vi "Digilens DLP Gen2 UI .vi"(11 "TopLevel In":refnum<class "TopLevel.lvclass">) -> (3 "TopLevel Out":refnum<class "TopLevel.lvclass">)   [LabVIEW 2022 SP3, in "TopLevel.lvclass"]
uses:
  TopLevel.lvclass
  Typedefs/SettinsgTabs--Tab.ctl
  Icons/Load.ctl
  Icons/HeadButton.ctl
  Icons/Enable.ctl
  Icons/go_button.ctl
  Typedefs/AdvPrinterControl--Tabs.ctl
  Common/Controls/ImageResolution--enum.ctl
  Icons/GreenControl_64.ctl
  GIS Printer/Typedefs/Print Types.ctl
  Typedefs/MainTabs--tabs.ctl
  Typedefs/Dummy--Tabs.ctl
  Typedefs/PurgeMode--Enum.ctl
  Typedefs/processMode--enum.ctl
  DAQWFE/LV_Source/Subsystems/DAQ/DAQ.lvclass
  <vilib>/TELLC/Dynamic CVT API/TD Dynamic CVT DVR--ref.ctl
  DAQWFE/LV_Source/Subsystems/DAQ/DataTypes/TD DAQ DI state change ev.ctl
  Typedefs/UserLevel_withoutNone--Enum.ctl
  DAQ_Common/DataTypes/TD IOCtrlUpdate.ctl
  DLP2/DLP2.lvclass/DLP2.ctl
  Typedefs/PrinterHeads--Enum.ctl
  Motor Controller/Typedefs/API Command Cluster.ctl
  Motor Controller/Typedefs/API Command Enum.ctl
  Motor Controller/Typedefs/SetExplicitMessage API Data.ctl
  Motor Controller/Typedefs/Motor Controller Parameter-Set.ctl
  IO/Typedefs/ICP1-D0 Channel Names.ctl
  Typedefs/HeadPrintData--Cluster.ctl
  Motor Controller/Typedefs/Motor Controller Parameter-Get.ctl
  Typedefs/API Command Enum.ctl
  Typedefs/PrimingMode APIData.ctl
  Typedefs/API Command Cluster.ctl
  GIS Printer/Typedefs/PrintCmdParameters--Cluster.ctl
  GIS Printer/Typedefs/IdlePrintCmdParameters--Cluster.ctl
  IO/Typedefs/ICP2-DO Channel Names.ctl
  GIS Printer/GIS Printer.lvclass/GIS Printer.ctl
  Common/Controls/RecipeInfo--Cluster.ctl
  Common/Controls/DLP RecipeTypesData--Cluster.ctl
  IO/IO.lvclass
  GIS Printer/GIS Printer.lvclass
  Motor Controller/Motor Controller.lvclass
  Motor Controller/Typedefs/Status.ctl
  Typedefs/Motor Controller Config Data.ctl
  Motor Controller/Typedefs/Stage Move Data.ctl
  Motor Controller/Typedefs/Batch Index Speed Data.ctl
  Motor Controller/Typedefs/Move Status.ctl
  IO/Typedefs/Pre Purge Parameters.ctl
  Database/Database.lvclass
  DLP2/DLP2.lvclass
  Common/Controls/TD MasterConfiguration DLPC2--cluster.ctl
  Common/Controls/DLPC2_Path--Cluster.ctl
  Common/Controls/TD HeadColorPaneMappingAll--cluster.ctl
  Common/Controls/TD HeadColorPaneMapping--cluster.ctl
  Typedefs/SpitVoltages--Cluster.ctl
  <vilib>/vision/Image Controls.llb/IMAQ Image.ctl
  Typedefs/TiffImageData--Cluster.ctl
  Common/Controls/Imageresolution--cluster.ctl
  GIS Printer/Typedefs/GIS Status--Cluster.ctl
  GIS Printer/Typedefs/HeadEnableStatus--cluster.ctl
  DLP2/DataTypes/SeperateLayersPython--cluster.ctl
  Common/Controls/PythonVersion--Enum.ctl
  Common/Controls/DLPConfig_RecipePrints.ctl
  Common/Controls/DLPConfig_CalibrationPrints.ctl
  Typedefs/LoginEventData--CLuster.ctl
  Typedefs/UserLevel--Enum.ctl
  Typedefs/printWeights--cluster.ctl
  DLP2/DataTypes/DLP2_PrinterHeadProperties.ctl
  Common/Controls/DLPConfig)Init_HeadPropertyAttr--Cluster.ctl
  Common/Controls/DLP_MaterialToHeadMapping--Cluster.ctl
  DLP2/DataTypes/DLP2_PrinterMaterialProperties.ctl
  Typedefs/InkIdleNodeConfigXML--Cluster.ctl
  IO/Typedefs/Status Cluster.ctl
  IO/Typedefs/ICP2-DI Channel Names.ctl
  IO/Typedefs/ICP1-AI Channel Names.ctl
  IO/Typedefs/ICP1-AO Channel Names.ctl
  IO/Typedefs/ICP2-AO Channel Names.ctl
  Motor Controller/Typedefs/Status_TopLevel--Cluster.ctl
  DLP2/DataTypes/LoadImagesData--cluster.ctl
  Common/Controls/RecipesFolderSummary--Cluster.ctl
  <vilib>/Analysis/baseanly.llb/Mean (DBL).vi
  DLP2/Accessors/Get PublicEvents.vi
  DAQWFE/LV_Source/DataTypes/GBL System.vi
  <vilib>/Utility/config.llb/Write Key (Path).vi
  GIS Printer/Methods/Variant_To_DVR.vi
  <userlib>/_OpenG.lib/array/array.llb/Sort 1D Array (I32)__ogtk.vi
  <vilib>/Analysis/NI_AALBase.lvlib
  <vilib>/Utility/config.llb/NI_LVConfig.lvlib
  <vilib>/vision/NI_Vision_Development_Module.lvlib
panel:
  in  "General":bool
  in  "CALIBRATION RECIPE XML FOLDER PATH":path
  in  "INITIALIZATION FILE PATH":path
  in  "PRODUCT RECIPE XML FOLDER PATH":path
  in  "Head 1 ColorPlane":u16(ring) items=["1", "0", "3", "2", "None", "None2"]
  in  "Head 2 ColorPlane":u16(ring) items=["1", "0", "3", "2", "None", "None2"]
  in  "Head 3 ColorPlane":u16(ring) items=["1", "0", "3", "2", "None", "None2"]
  in  "Head 4 ColorPlane":u16(ring) items=["1", "0", "3", "2", "None", "None2"]
  in  "Head 5 ColorPlane":u16(ring) items=["1", "0", "3", "2", "None", "None2"]
  in  "Head 6 ColorPlane":u16(ring) items=["1", "0", "3", "2", "None", "None2"]
  out "Head 1 Material":u16(ring) items=["109G", "113A_3", "507_2(50)", "507_2", "None", "None2"]
  out "Head 2 Material":u16(ring) items=["109G", "113A_3", "507_2(50)", "507_2", "None", "None2"]
  out "Head 3 Material":u16(ring) items=["109G", "113A_3", "507_2(50)", "507_2", "None", "None2"]
  out "Head 4 Material":u16(ring) items=["109G", "113A_3", "507_2(50)", "507_2", "None", "None2"]
  out "Head 5 Material":u16(ring) items=["109G", "113A_3", "507_2(50)", "507_2", "None", "None2"]
  out "Head 6 Material":u16(ring) items=["109G", "113A_3", "507_2(50)", "507_2", "None", "None2"]
  out "PPP search string":string
  in  "LoadImages":bool
  in  "Enable Disable With DO":T1
  in  "Jog (+) 1":bool
  in  "Jog (-) 1":bool
  in  "Abort 2":bool
  in  "Home 3":bool
  in  "Stage Abort":bool
  in  "Abort":bool
  in  "Home Stg 2":bool
  in  "Jog (+) 2":bool
  in  "Jog (-) 2":bool
  in  "Home":bool
  out "NameArray":string[](array[string])
  in  "INK H 11":T2
  out "LogINDetail":string
  in  "AdvPrinterTabsBtn":bool
  out "H6 Long Idle":bool
  out "H2 Long Idle":bool
  out "H1 Long Idle":bool
  out "H3 Long Idle":bool
  out "H4 Long Idle":bool
  out "H5 Long Idle":bool
  out "H6 Short Idle":bool
  out "H2 Short Idle":bool
  out "H1 Short Idle":bool
  out "H3 Short Idle":bool
  out "H4 Short Idle":bool
  out "H5 Short Idle":bool
  out "Stage Busy (Moves)":bool caption="Stage Busy"
  in  "5Pass":bool
  in  "10Pass":bool
  in  "Login":bool
  out "H6ColorPlane":string
  out "H5ColorPlane":string
  out "H4ColorPlane":string
  out "H3ColorPlane":string
  out "H2ColorPlane":string
  out "H1ColorPlane":string
  in  "IdleMode":T3
  in  "ImageResolution":T4
  out "Resolution":string
  in  "DLP GUI Config":path
  in  "SAVE DLP Config":bool
  in  "Apply DLP GUI Config":bool
  out "Meniscus Valve Open - R1_Status 2":T3
  out "Meniscus Valve Open - R2_Status 2":T3
  out "Meniscus Valve Open - R3_Status 2":T3
  out "Meniscus Valve Open - R4_Status 2":T3
  out "Meniscus Valve Open - R5_Status 2":T3
  out "Meniscus Valve Open - R6_Status 2":T3
  in  "PrinterControlsX":T5
  out "ImageMain":T6(plugin-control)
  in  "Head6 Temp 1":string
  in  "Head5 Temp 1":string
  in  "Head4 Temp 1":string
  in  "Head3 Temp 1":string
  in  "Head2 Temp 1":string
  in  "Head1 Temp 1":string
  in  "Stage Recipe XML File Path":path
  in  "Start":bool
  in  "Stage Move Status":i32(listbox)
  in  "Idle Intervals (s)":dbl=0.1
  in  "IdlePrint":bool
  in  "StartPrintSequence":bool
  in  "Load Customer Design":bool
  in  "Print Types":T7
  out "Version":string
  out "date/time string":string
  out "Type":string
  in  "GetMat&Color":bool
  in  "PPDuration (s)":dbl=3.0
  in  "Duration (s)":dbl=3.0
  out "AI ScanArray":dbl[](array[numeric])
  in  "Exit":bool
  in  "Settings":bool
  in  "Drop Watch":bool
  in  "Stage Control":bool
  in  "Printhead Service":bool
  in  "IPLC Process":bool
  out "Stage Busy Printer":bool caption="Busy"
  out "Status/Error :":string
  out "H 6":dbl
  out "H 5":dbl
  out "H 4":dbl
  out "H 3":dbl
  out "H 2":dbl
  out "H1":dbl
  in  "Tab Control":T8
  out "PrintStatus":string
  in  "Refresh Timer":bool
  out "HeadPrimeTimer":i32
  in  "Recipe":u16(ring) items=["c30v3_1 Recipe DOE485", "c30v3_1 Recipe DOE485 Green", "c30v3_1 Recipe PORtest"]
  in  "Product":u16(ring) items=["C30v3_1", "Haze", "SingleColor1_5"]
  in  "RecipeType":u16(ring) items=["PrintDesign", "Calibration"]
  in  "PrintControlTab":enum32{"Product", "Calibration"}(tab)
  in  "Print PPP Image":bool
  in  "RIP Recipe":bool
  out "CalPrint Counter":i32
  in  "Load Calibration Rx":bool
  in  "PrintHead Number":u16(ring)=1 caption="Head" items=["1", "2", "3", "4", "5", "6"]
  in  "Head Print Command":bool
  in  "Refresh":bool
  in  "PrimeHeads":bool
  in  "AbortPrinterOperation":bool
  out "ImageMain 5":T6(plugin-control)
  out "ImageMain 3":T6(plugin-control)
  out "ImageMain 4":T6(plugin-control)
  out "ImageMain 2":T6(plugin-control)
  in  "ProcessMode":T9
  in  "Load":T10
  in  "Laminate":T10
  in  "PurgeMove H1":T11
  in  "PurgeMove H2":T11
  in  "PurgeMove H3":T11
  in  "PurgeMove H4":T11
  in  "PurgeMove H5":T11
  in  "PurgeMove H6":T11
  out "Status":string
  in  "Jog (-)":bool
  in  "Jog (+)":bool
  in  "Jog Speed":i32
  in  "Print Speed (-)":bool
  in  "Print (+)":bool
  in  "Print Speed":i32
  in  "GoTo":i32
  in  "Speed":i32
  in  "Go":T12
  out "Position":dbl
  out "Pulse/mm":dbl
  in  "Head1":T11
  in  "Head2":T11
  in  "Head3":T11
  in  "Head4":T11
  in  "Head5":T11
  in  "Head6":T11
  in  "Read Status":bool
  in  "Enable Disable":T1
  in  "ClearStageAlarm":bool
  out "Stage Enabled":bool
  out "Stage Busy (Stage)":bool caption="Stage Busy"
  in  "PrinterControls 5":T2
  in  "Weights 5":dbl=0.15 min=0.01 max=0.15
  in  "Freq 5":i32
  in  "Head 5 Material 2":u16(ring) items=["109G", "113A_3", "507_2(50)", "507_2", "None", "None2"]
  in  "Heater-5 Off 2":bool
  out "Head 5 Act Temp":dbl
  in  "Enable Ink Ch-5":bool
  in  "Head5 TempSet":dbl
  in  "Head 5 Set":bool
  in  "Prime Mode 5":T13
  in  "Prime Duration 5":dbl=0.3
  in  "Prime Interavl 5":dbl
  in  "Prime Repeats 5":u8=1 min=1
  in  "StartPrime 5":bool
  in  "Stage Head5 2":bool
  out "H5 Status":T3
  out "HH5 Status":T3
  in  "PrinterControls 4":T2
  in  "Weights 4":dbl=0.15 min=0.01 max=0.15
  in  "Freq 4":i32
  in  "Head 4 Material 2":u16(ring) items=["109G", "113A_3", "507_2(50)", "507_2", "None", "None2"]
  in  "Heater-4 Off 2":bool
  out "Head 4 Act Temp":dbl
  in  "Enable Ink Ch-4":bool
  in  "Head4 TempSet":dbl
  in  "Head 4 Set":bool
  in  "Prime Mode 4":T13
  in  "Prime Duration 4":dbl=0.3
  in  "Prime Interval 4":dbl
  in  "Prime Repeats 4":u8=1 min=1
  in  "StartPrime 4":bool
  in  "Stage Head4 2":bool
  out "H4 Status":T3
  out "HH4 Status":T3
  in  "PrinterControls 6":T2
  in  "Weights 6":dbl=0.15 min=0.01 max=0.15
  in  "Freq 6":i32
  in  "Head 6 Material 2":u16(ring) items=["109G", "113A_3", "507_2(50)", "507_2", "None", "None2"]
  in  "Heater-6 Off 2":bool
  out "Head 6 Act Temp":dbl
  in  "Enable Ink Ch-6":bool
  in  "Head6 TempSet":dbl
  in  "Head 6 Set":bool
  in  "Prime Mode 6":T13
  in  "Prime Duration 6":dbl=0.3
  in  "Prime Interval 6":dbl
  in  "Prime Repeats 6":u8=1 min=1
  in  "StartPrime 6":bool
  in  "Stage Head6 2":bool
  out "H6 Status":T3
  out "HH6 Status":T3
  in  "PrinterControls 2":T2
  in  "Weights 2":dbl=0.15 min=0.01 max=0.15
  in  "Freq 2":i32=1
  in  "Head 2 Material 2":u16(ring) items=["109G", "113A_3", "507_2(50)", "507_2", "None", "None2"]
  in  "Heater-2 Off 2":bool
  out "Head 2 Act Temp":dbl
  in  "Enable Ink Ch-2":bool
  in  "Head2 TempSet":dbl
  in  "Head 2 Set":bool
  in  "StartPrime 2":bool
  in  "Prime Mode 2":T13
  in  "Prime Duration 2":dbl=0.3
  in  "Prime Interval 2":dbl=1.0
  in  "Prime Repeats 2":u8=1 min=1
  in  "Stage Head2 2":bool
  out "H2 Status":T3
  out "HH2 Status":T3
  in  "PrinterControls 3":T2
  in  "Weights 3":dbl=0.15 min=0.01 max=0.15
  in  "Freq 3":i32
  in  "Head 3 Material 2":u16(ring) items=["109G", "113A_3", "507_2(50)", "507_2", "None", "None2"]
  in  "Heater-3 Off 2":bool
  out "Head 3 Act Temp":dbl
  in  "Enable Ink Ch-3":bool
  in  "Head3 TempSet":dbl
  in  "Head 3 Set":bool
  in  "Prime Mode 3":T13
  in  "Prime Duration 3":dbl=0.3
  in  "Prime Interval 3":dbl
  in  "Prime Repeats 3":u8=1 min=1
  in  "StartPrime 3":bool
  in  "Stage Head3 2":bool
  out "H3 Status":T3
  out "HH3 Status":T3
  in  "PrinterControls":T2
  in  "Weights 1":dbl=0.15 min=0.01 max=0.15
  in  "Freq 1":i32=1
  in  "Head 1 Material 2":u16(ring) items=["109G", "113A_3", "507_2(50)", "507_2", "None", "None2"]
  in  "Heater-1 Off 2":bool
  in  "Enable Ink Ch-1":bool
  in  "Head1 TempSet":dbl
  in  "Head 1 Set":bool
  in  "Prime Mode 1":T13
  in  "Prime Duration 1":dbl=0.3
  in  "Prime Interval 1":dbl=1.0
  in  "Prime Repeats 1":u8=1 min=1
  in  "StartPrime 1":bool
  out "Head 1 Act Temp":dbl
  in  "Stage Head1 2":bool
  out "H1 Status":T3
  out "HH1 Status":T3
  in  "SaveINIXML":bool
  out "Counts":i32
  in  "Script CMD":bool
  in  "Digital IO":bool
  in  "Analog IO":bool
  out "SettingsTabs":T14
  out "SW - Ink Valve - R2":bool
  out "SW - Ink Valve - R1":bool
  out "SW - Ink Valve - R3":bool
  out "SW - Ink Valve - R4":bool
  out "SW - Ink Valve - R5":bool
  out "SW - Ink Valve - R6":bool
  out "SW - COVER INPUT SIDE":bool
  out "SW - COVER OUTPUT SIDE":bool
  out "SW - Purge - R2":bool
  out "SW - Purge - R1":bool
  out "SW - Purge - R3":bool
  out "SW - Purge - R4":bool
  out "SW - Purge - R5":bool
  out "SW - Purge - R6":bool
  in  "Dig H 1":T2
  in  "Meniscus Pressure Reg PWR - R1":bool
  in  "SW_LED - Ink Valve - R1":bool
  in  "Meniscus Valve Open - R1":bool
  out "Meniscus Valve Open - R1_Status":T3
  out "SW_LED - Ink Valve - R1_Status":T3
  out "Meniscus Pressure Reg PWR - R1_Status":T3
  in  "Dig H 2":T2
  in  "Meniscus Pressure Reg PWR - R2":bool
  in  "SW_LED - Ink Valve - R2":bool
  in  "Meniscus Valve Open - R2":bool
  out "Meniscus Pressure Reg PWR - R2_Status":T3
  out "SW_LED - Ink Valve - R2_Status":T3
  out "Meniscus Valve Open - R2_Status":T3
  in  "Dig H 3":T2
  in  "Meniscus Pressure Reg PWR - R3":bool
  in  "SW_LED - Ink Valve - R3":bool
  in  "Meniscus Valve Open - R3":bool
  out "Meniscus Pressure Reg PWR - R3_Status":T3
  out "SW_LED - Ink Valve - R3_Status":T3
  out "Meniscus Valve Open - R3_Status":T3
  in  "Dig H 4":T2
  in  "Meniscus Pressure Reg PWR - R4":bool
  in  "SW_LED - Ink Valve - R4":bool
  in  "Meniscus Valve Open - R4":bool
  out "Meniscus Pressure Reg PWR - R4_Status":T3
  out "SW_LED - Ink Valve - R4_Status":T3
  out "Meniscus Valve Open - R4_Status":T3
  in  "Dig H 5":T2
  in  "Meniscus Pressure Reg PWR - R5":bool
  in  "SW_LED - Ink Valve - R5":bool
  in  "Meniscus Valve Open - R5":bool
  out "Meniscus Pressure Reg PWR - R5_Status":T3
  out "SW_LED - Ink Valve - R5_Status":T3
  out "Meniscus Valve Open - R5_Status":T3
  in  "Dig H 6":T2
  in  "Meniscus Pressure Reg PWR - R6":bool
  in  "SW_LED - Ink Valve - R6":bool
  in  "Meniscus Valve Open - R6":bool
  out "Meniscus Pressure Reg PWR - R6_Status":T3
  out "SW_LED - Ink Valve - R6_Status":T3
  out "Meniscus Valve Open - R6_Status":T3
  in  "INK H 6":T2
  in  "Purge Valve Open - R6":bool
  in  "Recirc Pump On - R6":bool
  in  "Ink Flow Valve Open - R6":bool
  out "Purge Valve Open - R6_Status":T3
  out "Recirc Pump On - R6_Status":T3
  out "Ink Flow Valve Open - R6_Status":T3
  in  "INK H 5":T2
  in  "Purge Valve Open - R5":bool
  in  "Recirc Pump On - R5":bool
  in  "Ink Flow Valve Open - R5":bool
  out "Purge Valve Open - R5_Status":T3
  out "Recirc Pump On - R5_Status":T3
  out "Ink Flow Valve Open - R5_Status":T3
  in  "INK H 4":T2
  in  "Purge Valve Open - R4":bool
  in  "Recirc Pump On - R4":bool
  in  "Ink Flow Valve Open - R4":bool
  out "Purge Valve Open - R4_Status":T3
  out "Recirc Pump On - R4_Status":T3
  out "Ink Flow Valve Open - R4_Status":T3
  in  "INK H 3":T2
  in  "Purge Valve Open - R3":bool
  in  "Recirc Pump On - R3":bool
  in  "Ink Flow Valve Open - R3":bool
  out "Purge Valve Open - R3_Status":T3
  out "Recirc Pump On - R3_Status":T3
  out "Ink Flow Valve Open - R3_Status":T3
  in  "INK H 2":T2
  in  "Purge Valve Open - R2":bool
  in  "Recirc Pump On - R2":bool
  in  "Ink Flow Valve Open - R2":bool
  out "Purge Valve Open - R2_Status":T3
  out "Recirc Pump On - R2_Status":T3
  out "Ink Flow Valve Open - R2_Status":T3
  in  "INK H 1":T2
  in  "Purge Valve Open - R1":bool
  in  "Recirc Pump On - R1":bool
  in  "Ink Flow Valve Open - R1":bool
  out "Purge Valve Open - R1_Status":T3
  out "Recirc Pump On - R1_Status":T3
  out "Ink Flow Valve Open - R1_Status":T3
  in  "EnableHeadPrimeTimer":bool
  in  "MinCtrl 7":T2
  in  "Meniscus Vac Pump Speed-Set":bool
  in  "Meniscus Vac Pump Speed":dbl min=0.0 max=100.0
  in  "MinCtrl 4":T2
  in  "Meniscus Pressure Set - R4-Set":bool
  in  "Meniscus Pressure Set - R4":dbl min=0.0 max=20.0
  in  "MinCtrl 5":T2
  in  "Meniscus Pressure Set - R5-Set":bool
  in  "Meniscus Pressure Set - R5":dbl min=0.0 max=20.0
  in  "MinCtrl 6":T2
  in  "Meniscus Pressure Set - R6-Set":bool
  in  "Meniscus Pressure Set - R6":dbl min=0.0 max=20.0
  in  "MinCtrl 3":T2
  in  "Meniscus Pressure Set - R3-Set":bool
  in  "Meniscus Pressure Set - R3":dbl min=0.0 max=20.0
  in  "MinCtrl 2":T2
  in  "Meniscus Pressure Set - R2-Set":bool
  in  "Meniscus Pressure Set - R2":dbl min=0.0 max=20.0
  out "Meniscus Pressure Read - R1":dbl format="%#.2g"
  out "Meniscus Pressure Read - R2":dbl format="%#.2g"
  out "Meniscus Pressure Read - R3":dbl format="%#.2g"
  out "Meniscus Pressure Read - R4":dbl format="%#.2g"
  out "Meniscus Pressure Read - R5":dbl format="%#.2g"
  out "Meniscus Pressure Read - R6":dbl format="%#.2g"
  out "AI":bool
  in  "MinCtrl 1":T2
  in  "Meniscus Pressure Set - R1-Set":bool
  in  "Meniscus Pressure Set - R1":dbl min=0.0 max=20.0
  in  "SaveMeniscusinXML":bool
  in  "HomeOnComplete":bool
  out "Print #":i32=1 min=1 step=1
  in  "Print Passes":u8=1 min=1
  in  "Command File Path":path
  in  "TCP Commands & Responses":i32(listbox)
  in  "Print":bool
  in  "System Mode":u16(ring) items=["360dpi x 360dpi (1dpd) CMYK"]
  # "Color Plane Mapping"
  # "Material"
  # "Color Plane"
  # "Head-1"
  # "Head-2"
  # "Head-3"
  # "Head-4"
  # "Head-5"
  # "Head-6"
  # "%"
  # "%"
  # "Image"
  # "%"
  # "%"
  # "%"
  # "%"
  # "Jogging"
  # "SPIT"
  # "PURGE"
  # "HEAD"
  # "MATERIAL"
  # "WEIGHTS"
  # "INK CH ENBL"
  # "HEAT ENBL"
  # "ACTUAL(°C)"
  # "HEAD TEMP (°C)"
  # "Duration (s)"
  # "Interval (s)"
  # "Repeats"
  # "Frequency (Hz)"
  # "5"
  # "4"
  # "6"
  # "2"
  # "3"
  # "1"
  # "DO"
  # "Digital Inputs"
  # "Inch H2O"
  # "Inch H2O"
  # "Inch H2O"
  # "Inch H2O"
  # "Inch H2O"
  # "Inch H2O"
  # "%"
  # "Inch H2O"
  # "lnch H2O"
  # "Inch H2O"
  # "Inch H2O"
  # "Inch H2O"
  # "Inch H2O"
  # "Command Line Control"
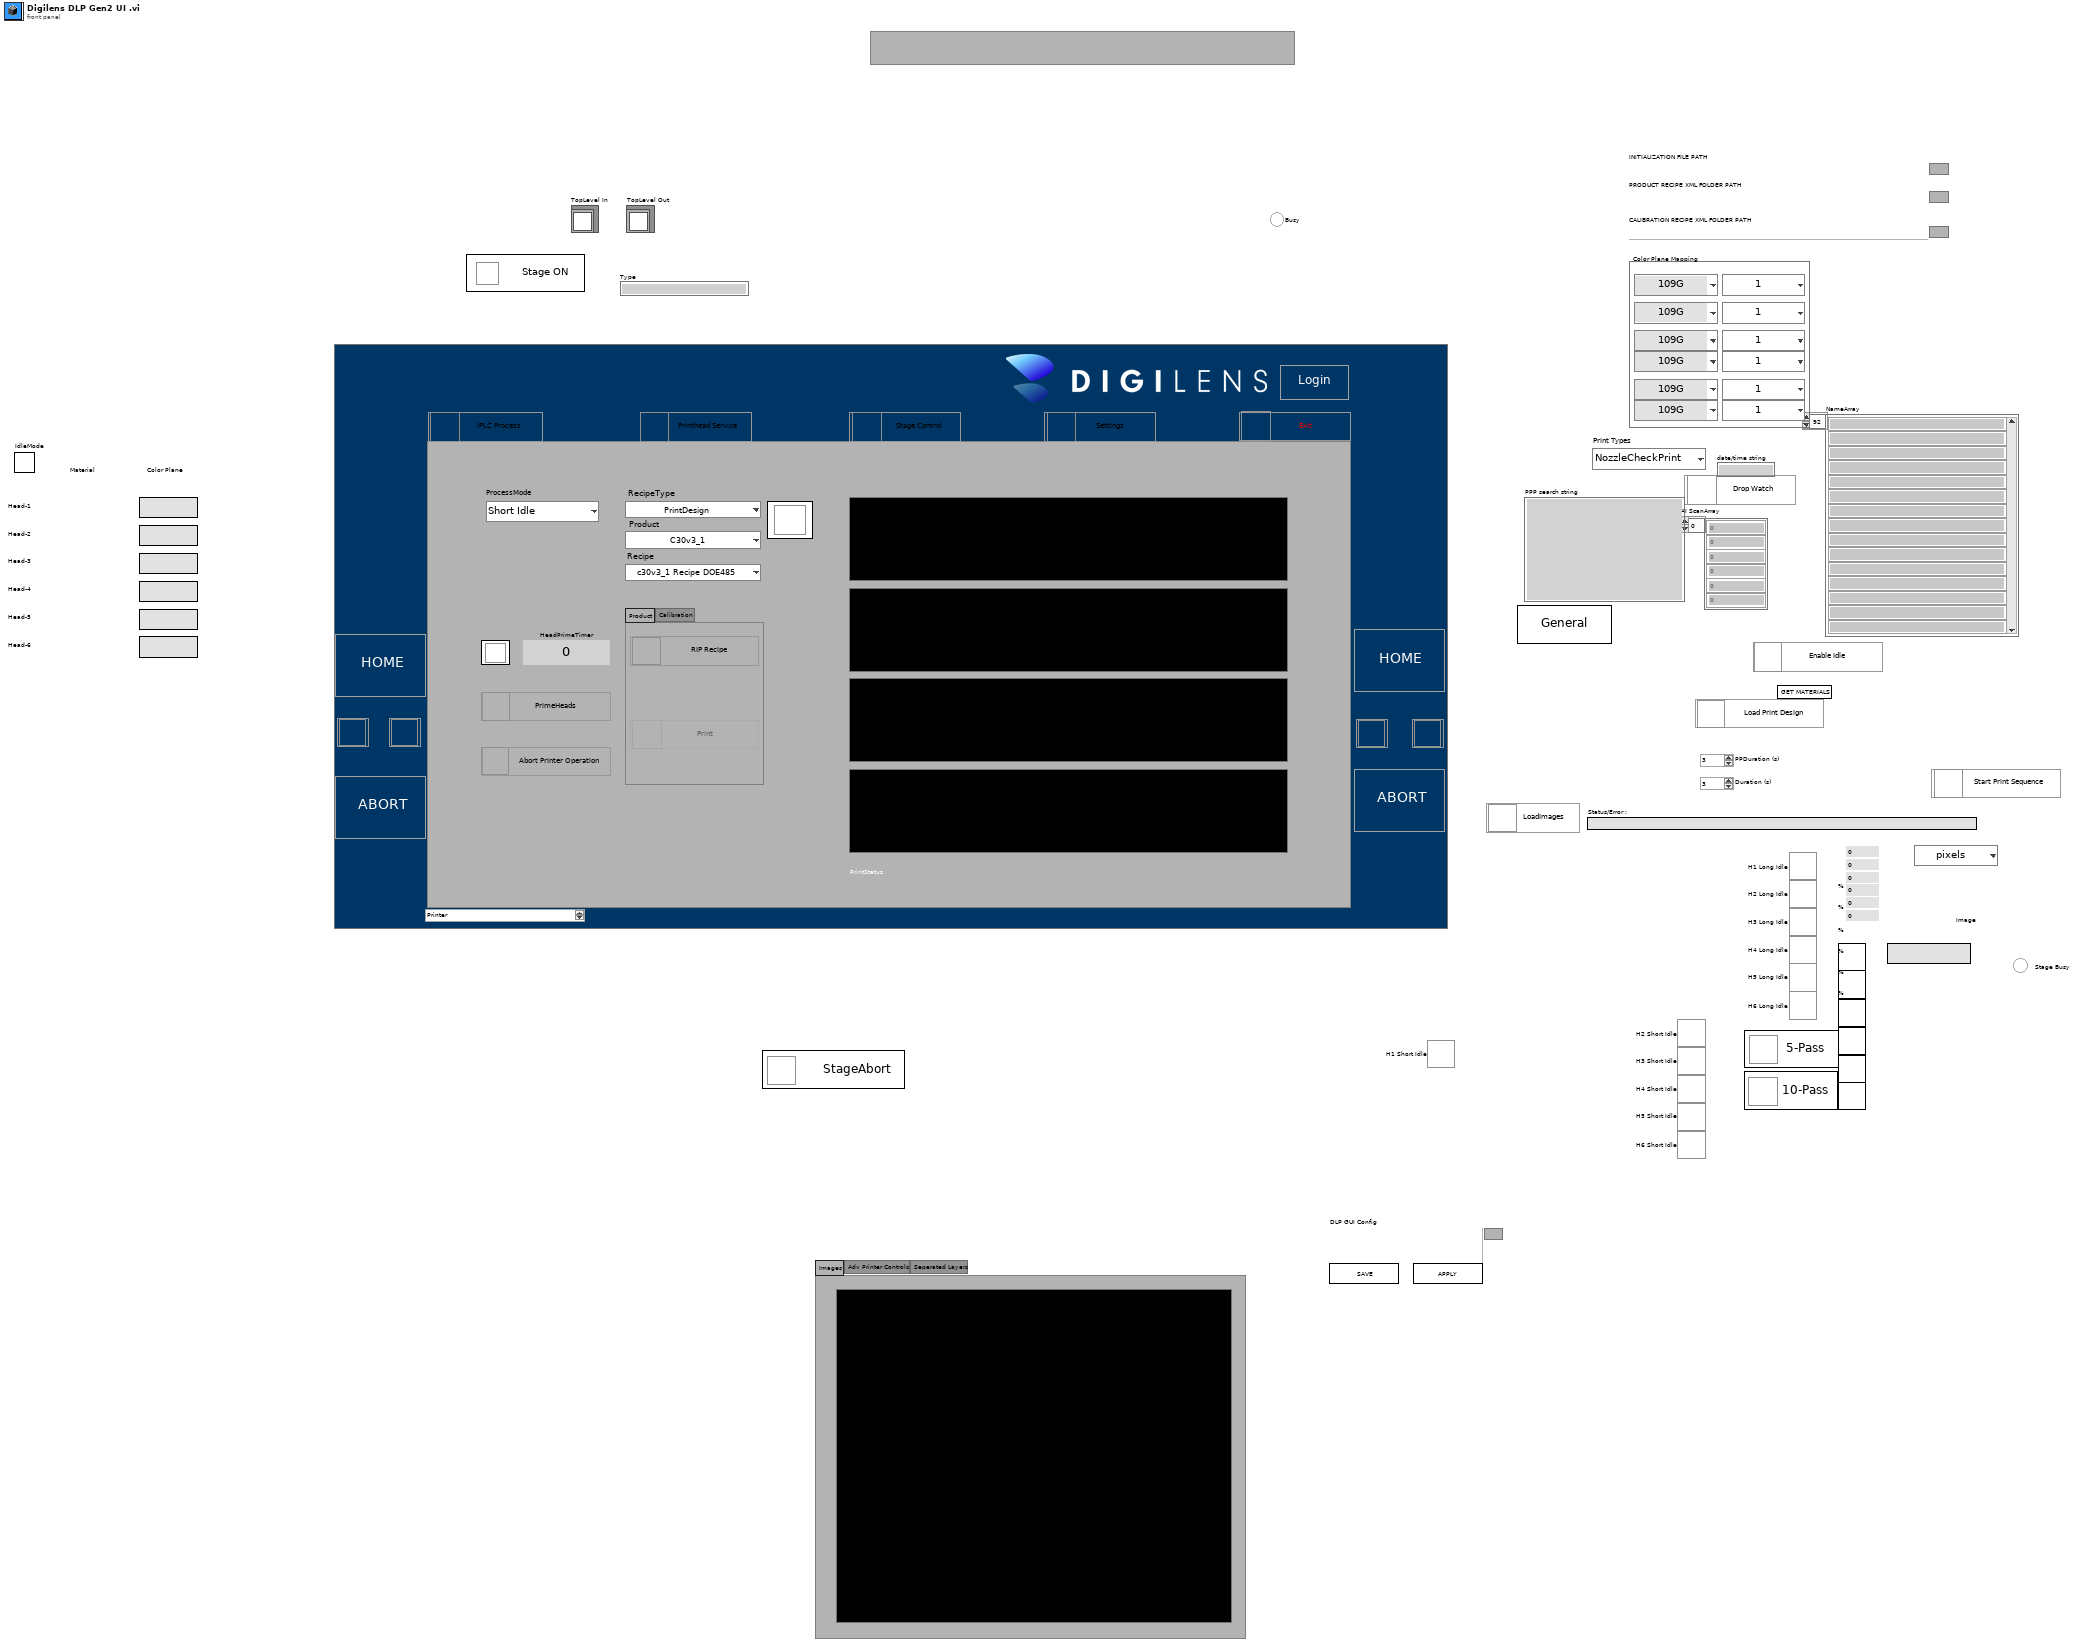
[diagram p1: front panel]
types:
  T1 = typedef "Enable.ctl" = bool
  T2 = typedef "Dummy--Tabs.ctl" = enum32{"Generic"}
  T3 = typedef "GreenControl_64.ctl" = bool
  T4 = typedef "ImageResolution--enum.ctl" = enum16{"pixels", "mm", "inches"}
  T5 = typedef "AdvPrinterControl--Tabs.ctl" = enum32{"Images", "Adv Printer Controls", "Seperated Layers"}
  T6 = typedef "IMAQ Image.ctl" = refnum<image>
  T7 = typedef "GIS Printer.lvclass/Print Types.ctl" = enum16{"NozzleCheckPrint", "StripWeightPrint", "PrintWeightPrint"}
  T8 = typedef "MainTabs--tabs.ctl" = enum32{"Printer", "Stage Control", "Purge and Prepurge", "Print Head Services", "Settings"}
  T9 = typedef "processMode--enum.ctl" = enum16{"Short Idle", "Long Idle ", "Process"}
  T10 = typedef "Load.ctl" = bool
  T11 = typedef "HeadButton.ctl" = bool
  T12 = typedef "go_button.ctl" = bool
  T13 = typedef "PurgeMode--Enum.ctl" = enum16{"Pre-Purge", "Purge", "Spit", "Shake"}
  T14 = typedef "SettinsgTabs--Tab.ctl" = enum32{"General", "Digital IO", "Analog IO", "Script CMD"}
  T15 = typedef "UserLevel_withoutNone--Enum.ctl" = enum16{"Engineer"}
  T16 = typedef "TD Dynamic CVT DVR--ref.ctl" = refnum<data-value>
  T17 = cluster{"String":string, "Response":refnum<user-event>, "Open":bool, "DAQ":refnum<class "DAQ.lvclass">, "DOStatus":T16, "DIStateChangeEv":refnum<user-event>, "RunningAvg WindowSize":i32, "AI Data":dbl[][]}
  T18 = typedef "PrinterHeads--Enum.ctl" = enum16{"-1", "1", "2", "3", "4", "5", "6"}
  T19 = typedef "IO.lvclass/ICP1-D0 Channel Names.ctl" = enum16{"None", "Meniscus Pressure Reg PWR - R1", "Meniscus Pressure Reg PWR - R2", "Meniscus Pressure Reg PWR - R3", "Meniscus Pressure Reg PWR - R4", "Meniscus Pressure Reg PWR - R5", "Meniscus Pressure Reg PWR - R6", "Clear Stage Alarm", "Servo ON", "Purge Valve Open - R1", "Purge Valve Open - R2", "Purge Valve Open - R3", "Purge Valve Open - R4", "Purge Valve Open - R5", "Purge Valve Open - R6"}
  T20 = typedef "Motor Controller.lvclass/SetExplicitMessage API Data.ctl" = cluster{"Motor Controller Parameter":T21, "value":i32}
  T21 = typedef "Motor Controller.lvclass/Motor Controller Parameter-Set.ctl" = enum16{"Print Speed", "Jog Speed", "PR Path", "Enable Servo", "Disable Servo", "Move Stage to Under PH1", "Move Stage to Under PH2", "Move Stage to Under PH3", "Move Stage to Under PH4", "Move Stage to Under PH5", "Move Stage to Under PH6", "Home Stage", "Return Stage to 0", "Print Stage", "Write Speed", "Write Index", "Stop Stage"}
  T22 = typedef "Motor Controller.lvclass/API Command Enum.ctl" = enum16{"GetExplicitMessage", "SetExplicitMessage", "Execute Stage Move Recipe", "Read Stage Move Recipe", "Abort"}
  T23 = typedef "Motor Controller.lvclass/API Command Cluster.ctl" = cluster{"Command":T22, "Arguments":string, "Data":variant}
  T24 = typedef "TopLevel.lvclass/HeadPrintData--Cluster.ctl" = cluster{"PrintImageFile":string, "PrintPass":u8, "EncoderSource":string, "PrintGoSource":string, "Head":T18}
  T25 = typedef "Motor Controller.lvclass/Motor Controller Parameter-Get.ctl" = enum16{"Print Speed", "Jog Speed", "PR Path", "Servo Enabled?"}
